vi "Enumeration Paths.vi"(8 "error in (no error)":errorcluster, 9 "Enumeration Name":string, 11 "LV-Protoc in":refnum<class "LV-Protoc.lvclass">) -> (0 "error out":errorcluster, 3 "LV-Protoc out":refnum<class "LV-Protoc.lvclass">, 4 "Built Enumeration":T1)   [LabVIEW 2020, in "LV-Protoc.lvlib" / "LV-Protoc.lvclass"]
uses:
  LV-Protoc.lvclass
  Enumeration Paths.ctl
  LV-Protoc.lvclass/LV-Protoc.ctl
  LV-Protoc.lvlib
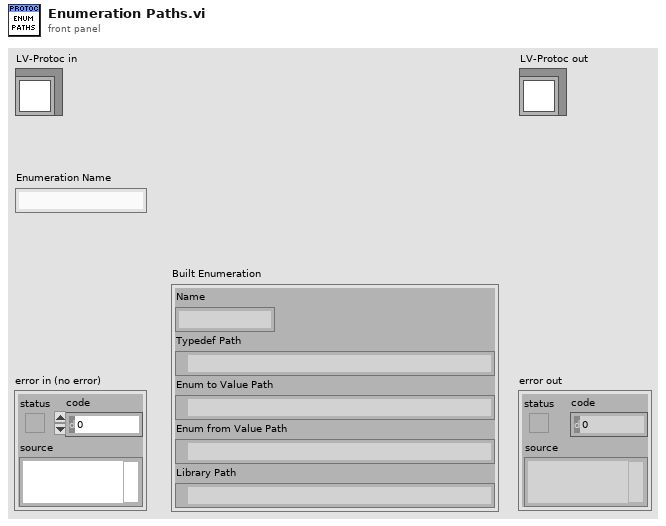
[diagram p1: front panel]
types:
  T1 = typedef "LV-Protoc.lvlib/Enumeration Paths.ctl" = cluster{"Name":string, "Typedef Path":path, "Enum to Value Path":path, "Enum from Value Path":path, "Library Path":path}
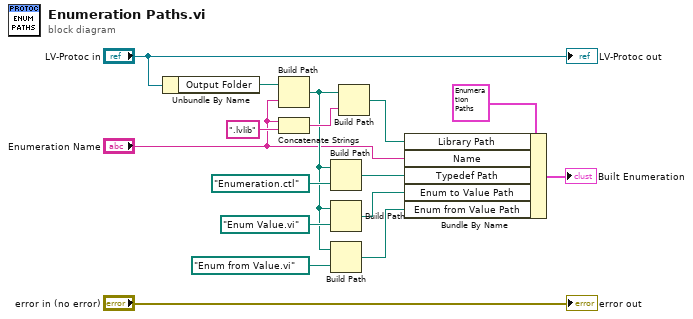
[diagram p0: block diagram]
diagram:
  n1 = Unbundle By Name("LV-Protoc in") -> ("Output Folder"=w16:path)
  n2 = Build Path(base path=w16, name or relative path="Enumeration Name") -> (appended path=w9:path)
  n3 = Concatenate Strings("Enumeration Name", ".lvlib" ("string")) -> (w14:string)
  n4 = Build Path(base path=w9, name or relative path=path "Enumeration.ctl") -> (appended path=w6:path)
  n5 = Build Path(base path=w9, name or relative path=path "Enum Value.vi") -> (appended path=w3:path)
  n6 = Build Path(base path=w9, name or relative path=path "Enum from Value.vi") -> (appended path=w2:path)
  n7 = Build Path(base path=w9, name or relative path=w14) -> (appended path=w5:path)
  n8 = Bundle By Name(cluster=T1 {"Name"="", "Typedef Path"=path "", "Enum to Value Path"=path "", "Enum from Value Path"=path "", "Library Path"=path ""} ("Built Enumeration"), "Library Path"=w5, "Name"="Enumeration Name", "Typedef Path"=w6, "Enum to Value Path"=w3, "Enum from Value Path"=w2) -> (→"Built Enumeration":T1)
  "error out" <- "error in (no error)"
  "LV-Protoc out" <- "LV-Protoc in"
